vi "Queue Reference (library variable).vi"() -> ()   [LabVIEW 2023, in "Error Manager.lvlib" / "New Error Window Loop Queue.lvclass"]
uses:
  Message (cluster).ctl
  Command (enum).ctl
  New Error Window Loop Queue.lvclass
panel:
  in  "Queue Reference":refnum<queue>
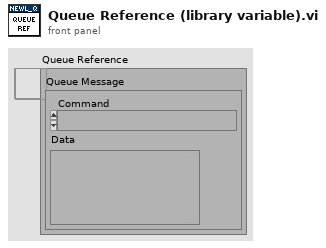
[diagram p1: front panel]
diagram:
